vi "svc_Get Window Info.vi"(8 "error in (no error)":errorcluster, 11 "scaled signal [EU]":waveform(dbl)={"t0"=timestamp(0 s since 1904-01-01), "dt"=0.0, "Y"=[]}) -> (0 "error out":errorcluster, 1 "window size":i32, 2 "window":T1 items=["Rectangle"=0, "Hanning"=1, "Hamming"=2, "Blackman-Harris"=3, "Exact Blackman"=4, "Blackman"=5, "Flat Top"=6, "4 Term B-Harris "=7, "7 Term B-Harris"=8, "Low Sidelobe"=9, "Blackman Nuttall"=11, "Triangle"=30, "Bartlett-Hanning"=31, "Bohman"=32, "Parzen"=33, "Welch"=34, "Kaiser"=60, "Dolph-Chebyshev"=61, "Gaussian"=62], 3 "dup scaled signal [EU]":waveform(dbl), 4 "window parameter":dbl)   [LabVIEW 2017]
uses:
  <vilib>/Analysis/4window.llb/windowTd.ctl
  <vilib>/Analysis/NI_AALPro.lvlib
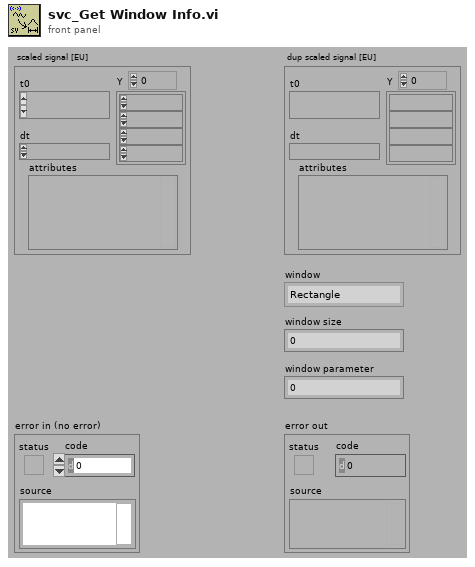
[diagram p1: front panel]
types:
  T1 = typedef "NI_AALPro.lvlib/windowTd.ctl" = u32
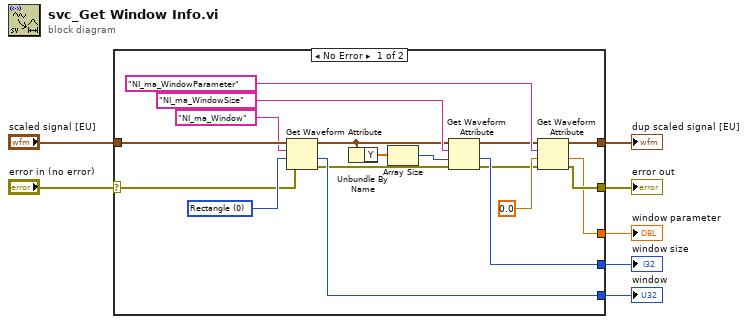
[diagram p0: block diagram]
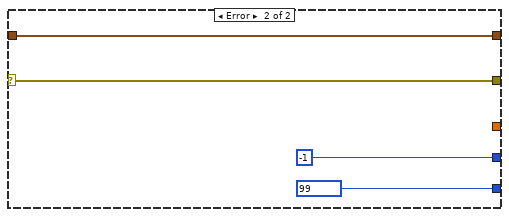
[diagram p2: hidden frame]
diagram:
  n1 = case shown="No Error" "error in (no error)" {
    selector: "error in (no error)" -> [w9 w29]
    tunnel: "scaled signal [EU]" -> [w25 w28]
    tunnel: [w21 w27] -> w2
    tunnel: [w10 w29] -> w6
    tunnel: [w13 w28] -> w5
    tunnel: [w20 -1] -> w3
    tunnel: [w8 _] -> w1
    frame No Error {
      w22 = T1 0 items=["Rectangle"=0, "Hanning"=1, "Hamming"=2, "Blackman-Harris"=3, "Exact Blackman"=4, "Blackman"=5, "Flat Top"=6, "4 Term B-Harris "=7, "7 Term B-Harris"=8, "Low Sidelobe"=9, "Blackman Nuttall"=11, "Triangle"=30, "Bartlett-Hanning"=31, "Bohman"=32, "Parzen"=33, "Welch"=34, "Kaiser"=60, "Dolph-Chebyshev"=61, "Gaussian"=62] ("window")
      n2 = Get Waveform Attribute(4:w9, 5:w22, 6:"NI_ma_Window" ("name"), 7:w25) -> (0:w16:errorcluster, 1:w21:T1, 3:w18:waveform(dbl))  [unwired: 1 out]
      n3 = Unbundle By Name ("Get Waveform Components")(w18) -> ("Y"=w19:dbl[])
      n4 = Array Size(array=w19) -> (size(s)=w17:i32)
      n5 = Get Waveform Attribute(4:w16, 5:w17, 6:"NI_ma_WindowSize" ("name"), 7:w18) -> (0:w11:errorcluster, 1:w20:i32, 3:w14:waveform(dbl))  [unwired: 1 out]
      n6 = Get Waveform Attribute(4:w11, 5:0.0, 6:"NI_ma_WindowParameter" ("name"), 7:w14) -> (0:w10:errorcluster, 1:w8:dbl, 3:w13:waveform(dbl))  [unwired: 1 out]
    }
    frame Error {
      w27 = T1 99 items=["Rectangle"=0, "Hanning"=1, "Hamming"=2, "Blackman-Harris"=3, "Exact Blackman"=4, "Blackman"=5, "Flat Top"=6, "4 Term B-Harris "=7, "7 Term B-Harris"=8, "Low Sidelobe"=9, "Blackman Nuttall"=11, "Triangle"=30, "Bartlett-Hanning"=31, "Bohman"=32, "Parzen"=33, "Welch"=34, "Kaiser"=60, "Dolph-Chebyshev"=61, "Gaussian"=62] ("window")
    }
  }
  "dup scaled signal [EU]" <- w5
  "error out" <- w6
  "window" <- w2
  "window size" <- w3
  "window parameter" <- w1
